vi "Integrator_v2.vi"(7 "median_w":T1, 9 "fs":dbl=119.0 format="%#_13g", 10 "Reset integrator":bool, 11 "Gyro data 3DOF":sgl[](array[numeric])) -> (0 "orientation":cluster{"Roll":dbl, "Pitch":dbl, "Yaw":dbl}, 1 "Yaw angle":dbl format="%#_5g", 2 "Pitch angle":dbl format="%#_5g", 3 "Roll angle":dbl format="%#_5g", 4 "offset removed w/ median":cluster{dbl, dbl, dbl})   [LabVIEW 2024]
uses:
  <vilib>/ptbypt/NI_PtbyPt.lvlib
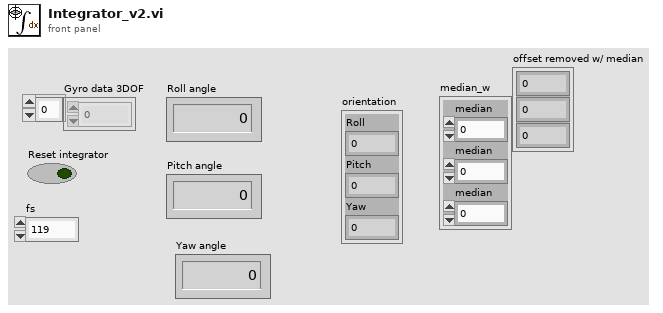
[diagram p1: front panel]
types:
  T1 = cluster{"median":dbl, "median":dbl, "median":dbl}
  T2 = cluster{"integral x(t)":dbl, "integral x(t)":dbl, "integral x(t)":dbl}
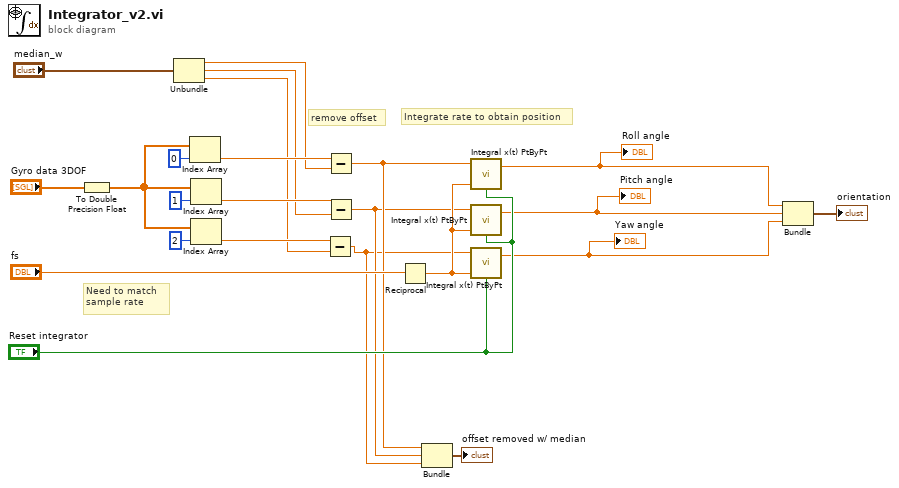
[diagram p0: block diagram]
diagram:
  # "remove offset"
  # "Need to match \nsample rate"
  # "Integrate rate to obtain position"
  n1 = To Double Precision Float(number="Gyro data 3DOF") -> (double precision float=w9:dbl[])
  n2 = Unbundle("median_w") -> ("median"=w10:dbl, "median"=w6:dbl, "median"=w5:dbl)
  n3 = Index Array "Index Array"(array=w9, index=0) -> (element=w11:dbl)
  n4 = Index Array(array=w9, index=1) -> (element=w8:dbl)
  n5 = Index Array(array=w9, index=2) -> (element=w7:dbl)
  n6 = Subtract(x=w7, y=w5) -> (x-y=w2:dbl)
  n7 = Subtract(x=w11, y=w10) -> (x-y=w4:dbl)
  n8 = Subtract(x=w8, y=w6) -> (x-y=w3:dbl)
  n9 = Reciprocal(x="fs") -> (1/x=w14:dbl)
  n10 = Bundle(w4, w3, w2) -> (→"offset removed w/ median":cluster{dbl, dbl, dbl})  [unwired: 1 in]
  n11 = call <vilib>:"Integral x(t) PtByPt.vi"("initialize"="Reset integrator", "dt"=w14, "x"=w4) -> ("integral x(t)"=w18:dbl)  [unwired: 1 in, 1 out]
  "Roll angle" <- w18
  n12 = call <vilib>:"Integral x(t) PtByPt.vi"("initialize"="Reset integrator", "dt"=w14, "x"=w3) -> ("integral x(t)"=w15:dbl)  [unwired: 1 in, 1 out]
  "Pitch angle" <- w15
  n13 = call <vilib>:"Integral x(t) PtByPt.vi"("initialize"="Reset integrator", "dt"=w14, "x"=w2) -> ("integral x(t)"=w16:dbl)  [unwired: 1 in, 1 out]
  "Yaw angle" <- w16
  n14 = Bundle "Bundle"("integral x(t)"=w18, "integral x(t)"=w15, "integral x(t)"=w16) -> (→"orientation":T2)  [unwired: 1 in]
